vi "Apply Settings.vi"(11 "Settings UI in":refnum<class "Settings UI.lvclass">) -> (3 "Settings UI out":refnum<class "Settings UI.lvclass">)   [LabVIEW 2020, in "Output Sequencer.lvlib" / "Settings UI.lvclass"]
uses:
  Settings UI.lvclass
  Settings UI.lvclass/Settings UI.ctl
  Globals/Dialog Strings.vi
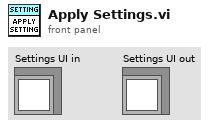
[diagram p1: front panel]
types:
  T1 = typedef "Output Sequencer.lvlib/Settings UI.lvclass/Settings.ctl" = cluster{"Plug-in Version":string, "Step Values":T2[], "Only Execute When Test Running":bool, "Reset Sequence When Test Starts":bool, "Number of Sequence Steps":i32, "Num of Analog Channels":i32, "Num of Digital Channels":i32, "Delay Before Starting Sequence":dbl, "Default Analog Values":dbl[], "Default Digital Values":bool[], "Max Iterations":u32, "Use last value when stopped":bool, "Prioritize exact values":bool, "Enable advanced step timing":bool, "Enable step conditions":bool, "Show confirmation dialogs":bool, "Start condition":string, "Enable re-triggering":bool, "Stop condition":string}
  T2 = typedef "Output Sequencer.lvlib/Settings UI.lvclass/Step Settings.ctl" = cluster{"Description":string, "Precondition":string, "Duration":dbl, "Mode":string, "Delay Between Values":dbl, "Analog Values":string[], "Digital Values":string[], "Postcondition":string, "On True":string, "On False":string}
  T3 = enum16{"Left Button", "Center Button", "Right Button", "Window Close"}
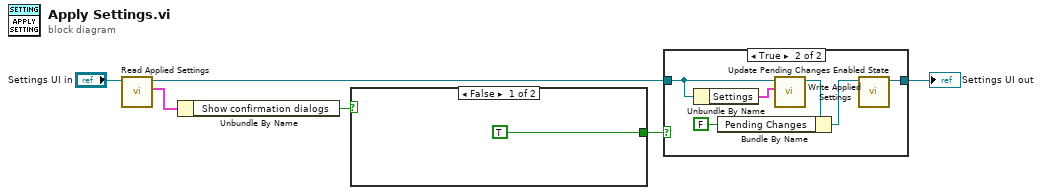
[diagram p0: block diagram]
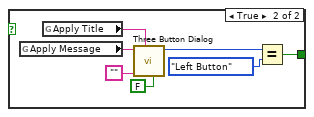
[diagram p2: hidden frame]
diagram:
  n1 = call "Read Applied Settings.vi"("UI Data in"="Settings UI in") -> ("Applied Settings"=w2:T1, "UI Data out"=w6:refnum<class "Settings UI.lvclass">)  [unwired: 8 in, 1 out]
  n2 = Unbundle By Name(w2) -> ("Show confirmation dialogs"=w3:bool)
  n3 = case shown="False" w3 {
    tunnel: [TRUE ("T button?") w14] -> w1
    frame False {
    }
    frame True {
      n4 = global read "Dialog Strings.vi" "Apply Message"() -> (w9:string)
      n5 = global read "Dialog Strings.vi" "Apply Title"() -> (w8:string)
      n6 = call <vilib>:"Three Button Dialog.vi"("Allow user to close window? (TRUE)"=FALSE, "Window Title (\"\")"=w8, "Right Button Text (\"Cancel\")"="", "message"=w9) -> ("Which Button?"=w11:T3)  [unwired: 7 in]
      n7 = Equal?(x=w11, y=T3."Left Button" ("Which Button?")) -> (x = y?=w14:bool)
    }
  }
  n8 = case shown="True" w1 {
    tunnel: w6 -> [w15 w21]
    tunnel: [w15 w16] -> w5
    frame False {
    }
    frame True {
      n9 = Unbundle By Name(w21) -> ("Settings"=w20:T1)
      n10 = call "Write Applied Settings.vi"("Applied Settings"=w20, "Settings UI in"=w21) -> ("Settings UI out"=w19:refnum<class "Settings UI.lvclass">)  [unwired: 8 in, 1 out]
      n11 = Bundle By Name(cluster=w19, "Pending Changes"=FALSE) -> (w17:refnum<class "Settings UI.lvclass">)
      n12 = call "Update Pending Changes Enabled State.vi"("UI Data in"=w17) -> ("UI Data out"=w16:refnum<class "Settings UI.lvclass">)  [unwired: 10 in]
    }
  }
  "Settings UI out" <- w5
